vi "BoolLight.vi"(0 "On":bool) -> ()   [LabVIEW 2014]
uses:
  <vilib>/Rock Robotics/WPI/Relay/WPI_RelayValue.ctl
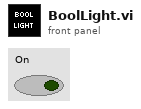
[diagram p1: front panel]
types:
  T1 = typedef "WPI_RelayDevRef.ctl" = cluster{"DevStatus":errorcluster, "Relay Channel":T2, "Controller":T3, "Relay Direction":T4}
  T2 = typedef "FPGA_DIORelayChannel.ctl" = enum8{"Relay 0", "Relay 1", "Relay 2", "Relay 3", "Invalid"}
  T3 = typedef "FPGA_TypedefDigitalModule.ctl" = enum16{"Controller 1"}
  T4 = typedef "WPI_RelayDirection.ctl" = enum16{"Both directions", "Forward only", "Reverse only"}
  T5 = typedef "WPI_RelayValue.ctl" = enum16{"Off", "On", "Forward", "Reverse"}
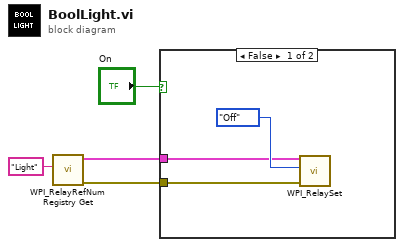
[diagram p0: block diagram]
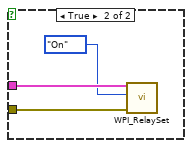
[diagram p2: hidden frame]
diagram:
  n1 = call <vilib>:"WPI_RelayRefNum Registry Get.vi"("refnum name"="Light") -> ("error out"=w1:errorcluster, "RelayDevRef"=w2:T1)  [unwired: 9 in]
  n2 = case shown="False" "On" {
    tunnel: w2 -> [w6 w10]
    tunnel: w1 -> [w5 w9]
    frame False {
      n3 = call <vilib>:"WPI_RelaySet.vi"("error in (no error)"=w5, "RelayValue"=WPI_RelayValue."Off", "RelayDevRef"=w6) -> ()  [unwired: 7 in, 2 out]
    }
    frame True {
      n4 = call <vilib>:"WPI_RelaySet.vi"("error in (no error)"=w9, "RelayValue"=WPI_RelayValue."On", "RelayDevRef"=w10) -> ()  [unwired: 7 in, 2 out]
    }
  }
